vi "DIMPowerSupply.set channel voltage.vi"(0 "i ref in":refnum<vi>, 2 "Voltage":dbl format="%.2f", 3 "ms timeout (10000)":i32=10000, 4 "channel":i32, 5 "error in (no error)":errorcluster) -> (14 "i ref out":refnum<vi>, 17 "timed out":bool, 19 "error out":errorcluster)   [LabVIEW 2014, in "DIMPowerSupply.lvlib"]
doc: "Sets the voltage by first converting the value to a raw voltage value and then writing the raw voltage value to DIM."
uses:
  DIMPowerSupply.lvlib
  CS_Core/CSSystem/CoreDefs/CoreDefs.error_type.ctl
  CS_Core/CSSystem/CoreDefs/CoreDefs.error_severity.ctl
  CS_Core/CSApplicationBaseClasses/PSChannelBase/PSChannelBase.directionType.ctl
  CS_Core/CSApplicationBaseClasses/PSChannelBase/PSChannelBase.serviceType.ctl
  CSlibraries/UtilityLib/UtilityLib.valueStatus.ctl
  CS_Core/CSSystem/CoreLib/CoreLib.lvlib
  CSlibraries-extern/DimLVEvent/LVDimInterface/LVDimInterface.lvlib
  CS_Core/CSApplicationBaseClasses/PSChannelBase/PSChannelBase.lvlib
  CSlibraries/UtilityLib/UtilityLib.lvlib
  CS_Core/CSApplicationBaseClasses/DeviceBase/DeviceBase.lvlib
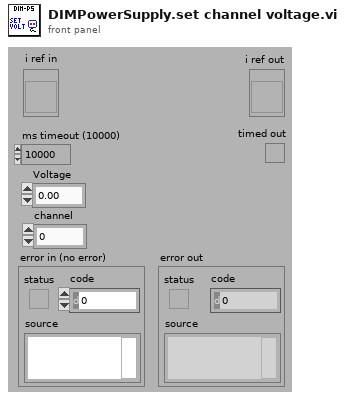
[diagram p1: front panel]
types:
  T1 = typedef "CoreDefs.error_severity.ctl" = enum16{"undefined", "information", "warning", "error", "fatal"}
  T2 = typedef "CoreDefs.error_type.ctl" = enum16{"no error", "can't load process", "can't unload process", "process does not exist", "can't install process", "can't remove process", "unknown function", "time out", "can't execute function", "duplicate queue name", "super not found", "caller queue invalid", "can't ping process", "unknown error", "VISA Error", "VISA timeout", "GPIB timeout", "GPIB error", "communication error", "data type mismatch", "can't read data from OPC server", "can't write data to OPC server", "OET error", "function not implemented", "process already exists", "invalid Shared Variable name", "error writing Shared Variable", "error reading Shared Variable", "invalid client name", "corrupt database", "unknown class", "call not authorized", "parameter out of range", "OET timeout: can't get data to modify", "invalid queue name", "requested operation incompatible with current state", "event undefined", "event disabled", "state undefined", "caller is not a friend", "EventBuilder: bad eventID", "EventBuilder: no DAQ devices", "a thread must not stop itself", "UNUSED ELEMENT4", "DiscArchiver: eventData incomplete", "DiscArchiver: eventData does not belong to run", "DiscArchiver: can't open file", "DiscArchiver: can't write to file", "DiscArchiver: available disc space low", "can't acquire semaphore", "error reading data from database", "notifier object is not existing", "can't register process", "can't unregister process", "illegal event type", "object disabled", "object already exists", "can't change state", "Instrument not found", "no connection to remote node", "invalid reference", "N/A", "UNUSED ELEMENT 1", "element not found", "illegal TCP/IP connection detected", "object does not exist", "invalid access ID", "unknown CS system", "invalid privilige", "unsupported data type", "unsupported server type", "IO server already exists", "Shared Variable already exists"}
  T3 = typedef "UtilityLib.lvlib/UtilityLib.valueStatus.ctl" = enum16{"no info available", "stand by/off", "on", "warning", "alarm/malfunction", "not implemented", "user action required", "important information", "system default", "control default", "indicator default", "button default"}
  T4 = typedef "PSChannelBase.lvlib/PSChannelBase.serviceType.ctl" = enum16{"onOff", "voltage", "current", "tripCurrent", "rampUpSpeed", "rampDownSpeed", "status"}
  T5 = typedef "PSChannelBase.lvlib/PSChannelBase.directionType.ctl" = enum16{"unknown", "update actual value", "update nominal value", "update both"}
  T6 = typedef "DIMPowerSupply.lvlib/DIMPowerSupply.ranges type.ctl" = cluster{"deviceMin":dbl, "deviceMax":dbl, "numberMin":u16, "numberMax":u16, "U16?":bool, "factor":dbl}
  T7 = typedef "DIMPowerSupply.lvlib/DIMPowerSupply.i attribute.ctl" = cluster{"ctrlValueID":i32}
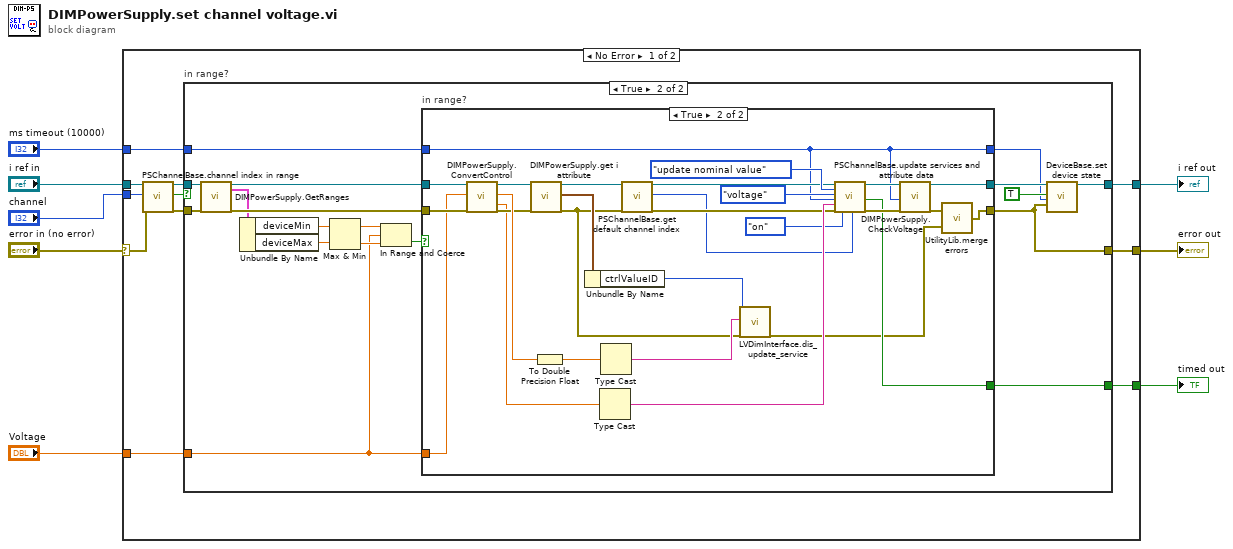
[diagram p0: block diagram]
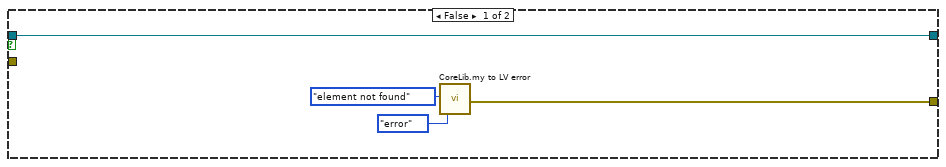
[diagram p2: hidden frame]
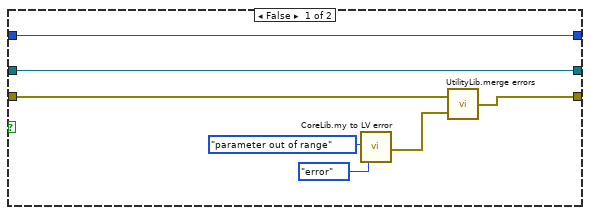
[diagram p3: hidden frame]
diagram:
  n1 = case shown="No Error" "error in (no error)" {
    selector: "error in (no error)" -> [w10 w77]
    tunnel: [w19 w77] -> w8
    tunnel: [w18 w78] -> w7
    tunnel: [w17 _] -> w6
    tunnel: "ms timeout (10000)" -> [w16 _]
    tunnel: "i ref in" -> [w14 w78]
    tunnel: "Voltage" -> [w15 _]
    tunnel: "channel" -> [w12 _]
    frame No Error {
      n2 = call "PSChannelBase.channel index in range.vi"("i ref in"=w14, "channelIndex"=w12, "error in (no error)"=w10) -> ("i ref out"=w13:refnum<vi>, "in range"=w11:bool, "error out"=w9:errorcluster)  [unwired: 14 in]
      n3 = case "in range?" shown="True" w11 {
        tunnel: [w22 w25] -> w19
        tunnel: [w23 w24] -> w18
        tunnel: [_ w41] -> w17
        tunnel: w16 -> [_ w40]
        tunnel: w13 -> [w23 w39]
        tunnel: w15 -> [_ w31]
        tunnel: w9 -> [_ w29]
        frame False {
          n4 = call "CoreLib.my to LV error.vi"("ErrorTypes"=CoreDefs.error_type."element not found", "severityLevel"=CoreDefs.error_severity."error") -> ("myErrorCluster"=w22:errorcluster)  [unwired: 16 in, 1 out]
        }
        frame True {
          n5 = call "DIMPowerSupply.GetRanges.vi"("i ref in"=w39, "error in (no error)"=w29) -> ("i ref out"=w38:refnum<vi>, "ControlRanges"=w36:T6, "error out"=w37:errorcluster)  [unwired: 14 in, 1 out]
          n6 = Unbundle By Name(w36) -> ("deviceMin"=w35:dbl, "deviceMax"=w34:dbl)
          n7 = Max & Min(x=w35, y=w34) -> (max(x,y)=w33:dbl, min(x,y)=w32:dbl)
          n8 = In Range and Coerce(upper limit=w33, x=w31, lower limit=w32) -> (In Range?=w30:bool)  [unwired: 1 out]
          n9 = case "in range?" shown="True" w30 {
            tunnel: [w42 w49] -> w25
            tunnel: [w47 w53] -> w27
            tunnel: [_ w64] -> w41
            tunnel: w40 -> [w45 w52]
            tunnel: w38 -> [w47 w76]
            tunnel: w37 -> [w43 w75]
            tunnel: w31 -> [_ w74]
            tunnel: [w45 w52] -> w26
            frame False {
              n10 = call "CoreLib.my to LV error.vi"("ErrorTypes"=CoreDefs.error_type."parameter out of range", "severityLevel"=CoreDefs.error_severity."error") -> ("myErrorCluster"=w44:errorcluster)  [unwired: 16 in, 1 out]
              n11 = call "UtilityLib.merge errors.vi"("error2 (no error)"=w44, "error1 (no error)"=w43) -> ("error out"=w42:errorcluster)
            }
            frame True {
              n12 = call "DIMPowerSupply.ConvertControl.vi"("i ref in"=w76, "nominal PS voltage [V]"=w74, "error in (no error)"=w75) -> ("i ref out"=w71:refnum<vi>, "nominal module value"=w72:dbl, "nominal module voltage [V]"=w61:dbl, "error out"=w70:errorcluster)  [unwired: 13 in]
              n13 = call "DIMPowerSupply.get i attribute.vi"("i ref in"=w71, "error in (no error)"=w70) -> ("i ref out"=w58:refnum<vi>, "i attribute"=w73:T7, "error out"=w57:errorcluster)  [unwired: 15 in]
              n14 = To Double Precision Float(number=w72) -> (double precision float=w67:dbl)
              n15 = Unbundle By Name(w73) -> ("ctrlValueID"=w69:i32)
              n16 = Type Cast(x=w61) -> (*(type *) &x=w60:string)  [unwired: 1 in]
              n17 = Type Cast(x=w67) -> (*(type *) &x=w68:string)  [unwired: 1 in]
              n18 = call "PSChannelBase.get default channel index.vi"("i ref in"=w58, "error in (no error)"=w57) -> ("i ref out"=w56:refnum<vi>, "defaultChannelIndex"=w54:i32, "error out"=w55:errorcluster)  [unwired: 15 in]
              n19 = call "LVDimInterface.dis_update_service.vi"("my_serviceID"=w69, "data"=w68, "error in (no error)"=w57) -> ("error out"=w50:errorcluster)  [unwired: 14 in, 2 out]
              n20 = call "PSChannelBase.update services and attribute data.vi"("i ref in"=w56, "direction"=PSChannelBase.directionType."update nominal value", "service"=PSChannelBase.serviceType."voltage", "ms timeout (10000)"=w52, "value"=w60, "error in (no error)"=w55, "quality"=UtilityLib.valueStatus."on", "channelNumber"=w54) -> ("i ref out"=w66:refnum<vi>, "timed out"=w64:bool, "error out"=w65:errorcluster)  [unwired: 9 in]
              n21 = call "DIMPowerSupply.CheckVoltage.vi"("i ref in"=w66, "ms timeout (10000)"=w52, "error in (no error)"=w65) -> ("i ref out"=w53:refnum<vi>, "error out"=w51:errorcluster)  [unwired: 14 in, 1 out]
              n22 = call "UtilityLib.merge errors.vi"("error2 (no error)"=w50, "error1 (no error)"=w51) -> ("error out"=w49:errorcluster)
            }
          }
          n23 = call "DeviceBase.set device state.vi"("i ref in"=w27, "implicit"=TRUE, "ms timeout (10000)"=w26, "device error"=w25) -> ("i ref out"=w24:refnum<vi>)  [unwired: 13 in, 2 out]
        }
      }
    }
    frame Error {
    }
  }
  "error out" <- w8
  "i ref out" <- w7
  "timed out" <- w6
